vi "OpenDotNetReferenceInArray.vi"(2 "Double Num":dbl=7.3, 3 "Integer Num":i32=7, 4 "String Value":string) -> (0 "error out":errorcluster, 1 "Array Of .NET Refs":refnum<k24>[](array[refnum]))   [LabVIEW 2010]
uses:
  \\camila\f$/Tests/LVBuildValidation/10.0/Automated/FlexLVAdapter30/Refnums/DotNetRefnum/LabviewDNTest.dll
  LabviewDNTest.dll
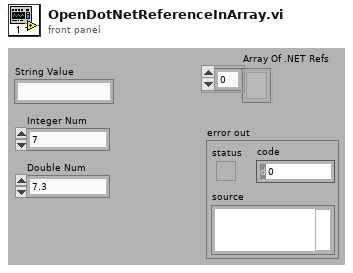
[diagram p1: front panel]
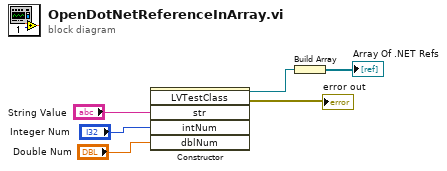
[diagram p0: block diagram]
diagram:
  n1 = constructor class="LVTestClass"("str"="String Value", "intNum"="Integer Num", "dblNum"="Double Num") -> (reference out=w1:refnum<k24>, error out=→"error out":errorcluster)  [unwired: 3 in, 4 out]
  n2 = Build Array(w1) -> (→"Array Of .NET Refs":refnum<k24>[])
